vi "measure_cnt.vi"(8 "error in (no error)":errorcluster, 11 "datalog path (use dialog)":path) -> (0 "error out":errorcluster, 3 "msr cnt":dbl)   [LabVIEW 2013]
uses:
  <vilib>/regexp/Match Regular Expression.xnode
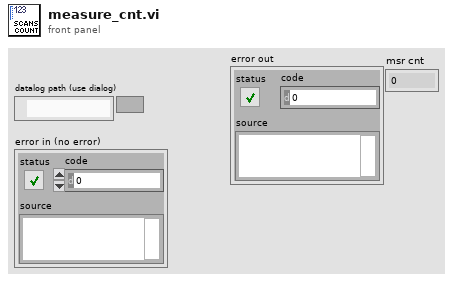
[diagram p1: front panel]
types:
  T1 = enum16{"open", "replace", "create", "open or create", "replace or create", "replace or create with confirmation"}
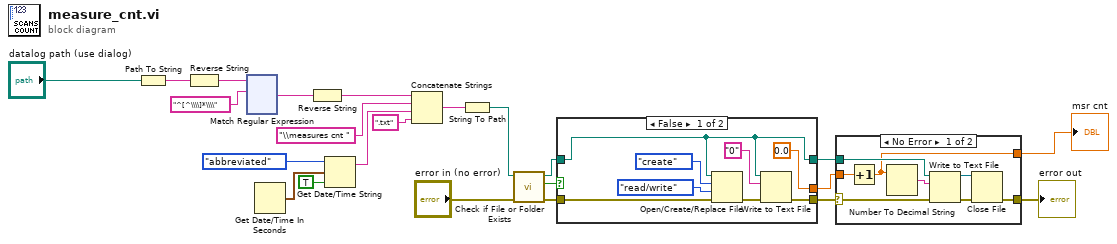
[diagram p0: block diagram]
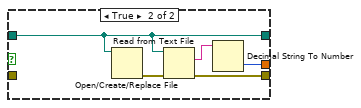
[diagram p2: hidden frame]
diagram:
  n1 = Path To String(path="datalog path (use dialog)") -> (string=w6:string)
  n2 = Reverse String(1:w6) -> (0:w8:string)
  n3 = xnode "Match Regular Expression"("input string"=w8, "regular expression"="^[^\\\\]*\\\\") -> ("after match"=w9:string)  [unwired: 4 in, 4 out]
  n4 = Get Date/Time In Seconds() -> (seconds since 1Jan1904=w14:timestamp)
  n5 = Reverse String(1:w9) -> (0:w10:string)
  n6 = Get Date/Time String(date format (0)=enum16{"short", "long", "abbreviated"}."abbreviated", seconds (now)=w14, want seconds? (F)=TRUE) -> (date string=w15:string)  [unwired: 1 out]
  n7 = Concatenate Strings(w10, "\\measures cnt " ("string"), w15, ".txt" ("string")) -> (w5:string)
  n8 = String To Path(string=w5) -> (path=w18:path)
  n9 = call <vilib>:"Check if File or Folder Exists.vi"("error in (no error)"="error in (no error)", "path"=w18) -> ("error out"=w20:errorcluster, "file or folder exists?"=w16:bool, "dup path"=w17:path)  [unwired: 7 in]
  n10 = case shown="False" w16 {
    tunnel: w17 -> [w24 w32]
    tunnel: [0.0 ("appr") w35] -> w22
    tunnel: [w26 w34] -> w19
    tunnel: w20 -> [w27 _]
    tunnel: [w24 w32] -> w23
    frame False {
      n11 = Open/Create/Replace File(file path (use dialog)=w24, error in=w27, operation (0:open)=T1."create", access (0:read/write)=enum16{"read/write", "read-only", "write-only"}."read/write") -> (error out=w29:errorcluster)  [unwired: 2 in, 2 out]
      n12 = Write to Text File(file (use dialog)=w24, text="0", error in=w29) -> (error out=w26:errorcluster)  [unwired: 1 in, 2 out]
    }
    frame True {
      n13 = Open/Create/Replace File(file path (use dialog)=w32) -> (error out=w33:errorcluster)  [unwired: 5 in, 2 out]
      n14 = Read from Text File(file (use dialog)=w32, error in=w33) -> (text=w36:string, error out=w34:errorcluster)  [unwired: 2 in, 2 out]
      n15 = Decimal String To Number(string=w36) -> (number=w35:i32)  [unwired: 2 in, 1 out]
    }
  }
  n16 = case shown="No Error" w19 {
    selector: w19 -> [w40 w46]
    tunnel: w22 -> [w44 w45]
    tunnel: w23 -> [w39 _]
    tunnel: [w38 w46] -> w2
    tunnel: [w37 w45] -> w1
    frame No Error {
      n17 = Increment(x=w44) -> (x+1=w37:dbl)
      n18 = Number To Decimal String(number=w37) -> (decimal integer string=w43:string)  [unwired: 1 in]
      n19 = Write to Text File(file (use dialog)=w39, text=w43, error in=w40) -> (refnum out=w42:refnum<file>, error out=w41:errorcluster)  [unwired: 1 in, 1 out]
      n20 = Close File(refnum=w42, error in=w41) -> (error out=w38:errorcluster)  [unwired: 1 out]
    }
    frame Error {
    }
  }
  "error out" <- w2
  "msr cnt" <- w1
